vi "VNA and Keithlay 2400.vi"() -> ()   [LabVIEW 2022 SP3]
uses:
  <instrlib>/Keithley 24XX/Public/Data/Read (Single Point).vi
  <vilib>/Utility/file.llb/Write Delimited Spreadsheet (DBL).vi
  <instrlib>/Keithley 24XX/Keithley 24XX.lvlib
  Agilent ENA Series/Agilent ENA Series.lvlib
panel:
  out "Numeric 3":dbl
  in  "Numeric 2":dbl
  in  "Numeric":i32
  out "Status":sgl
  out "Current":sgl
  out "XY Graph":cluster{dbl[], "Primary / Real":dbl[]}(graph)
  out "Step V":dbl
  in  "Points (>1) V":u32=66
  in  "End V":dbl
  in  "Start V":dbl=-3.0
  in  "VNA VISA resource name":refnum<visa-resource-name>="E5061A"
  in  "Port ( 1)":i32=1
  in  "Measurement Parameters":u16(ring)=1 items=["S11", "S21", "S31", "S41", "S12", "S22", "S32", "S42", "S13", "S23", "S33", "S43", "S14", "S24", "S34", "S44", "A", "B", "C", "D", "R1", "R2", "R3", "R4"]
  in  "Power Level (dBm)":dbl=-5.0 format="%^.2g"
  in  "VNA Points":i32=1000
  in  "Start (Mhz)":dbl=1.0 format="%^.2e"
  in  "Stop (MHz)":dbl=10.0 format="%^.2e"
  in  "Trigger Source":u16(ring) items=["Internal", "External", "Manual", "BUS"]
  in  "Point Trigger (F: Disable)":bool
  in  "Continuous Sweep (T: Enable)":bool=TRUE
  in  "Averaging State (F: Off)":bool
  in  "Average Factor (16)":i32=16
  in  "IF Bandwidth (100000.0)":dbl=1000.0 format="%^.1e"
  in  "Smoothing State (F: Off)":bool
  in  "Wait time (ms)":dbl=4000.0
  in  "file path (dialog if empty)":path=path "C:/Users/B1172_SHG/Documents/NOEMS/test.txt"
  in  "Output Type  (0: Immediate)":u16(ring) items=["Immediate", "Triggered"]
  in  "Source Mode  (0: Voltage)":u16(ring) items=["Voltage", "Current"]
  out "Current Voltage":dbl
  in  "Compliance  Level (0.1)":dbl=0.1
  in  "Keithley VISA resource name":refnum<visa-resource-name>
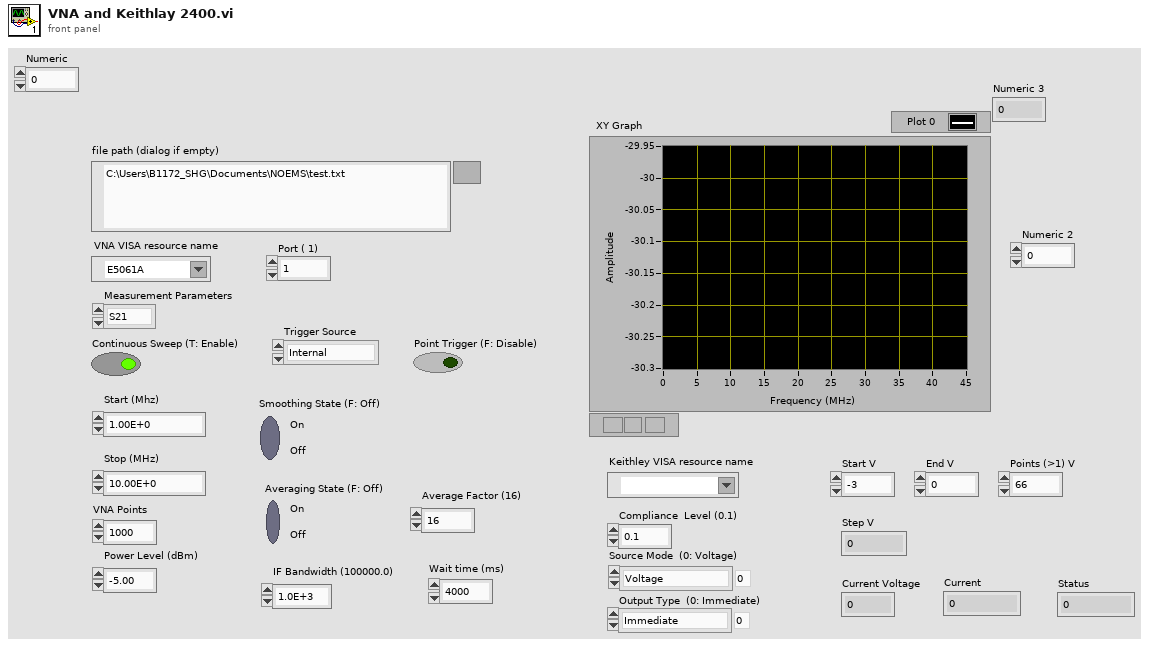
[diagram p1: front panel]
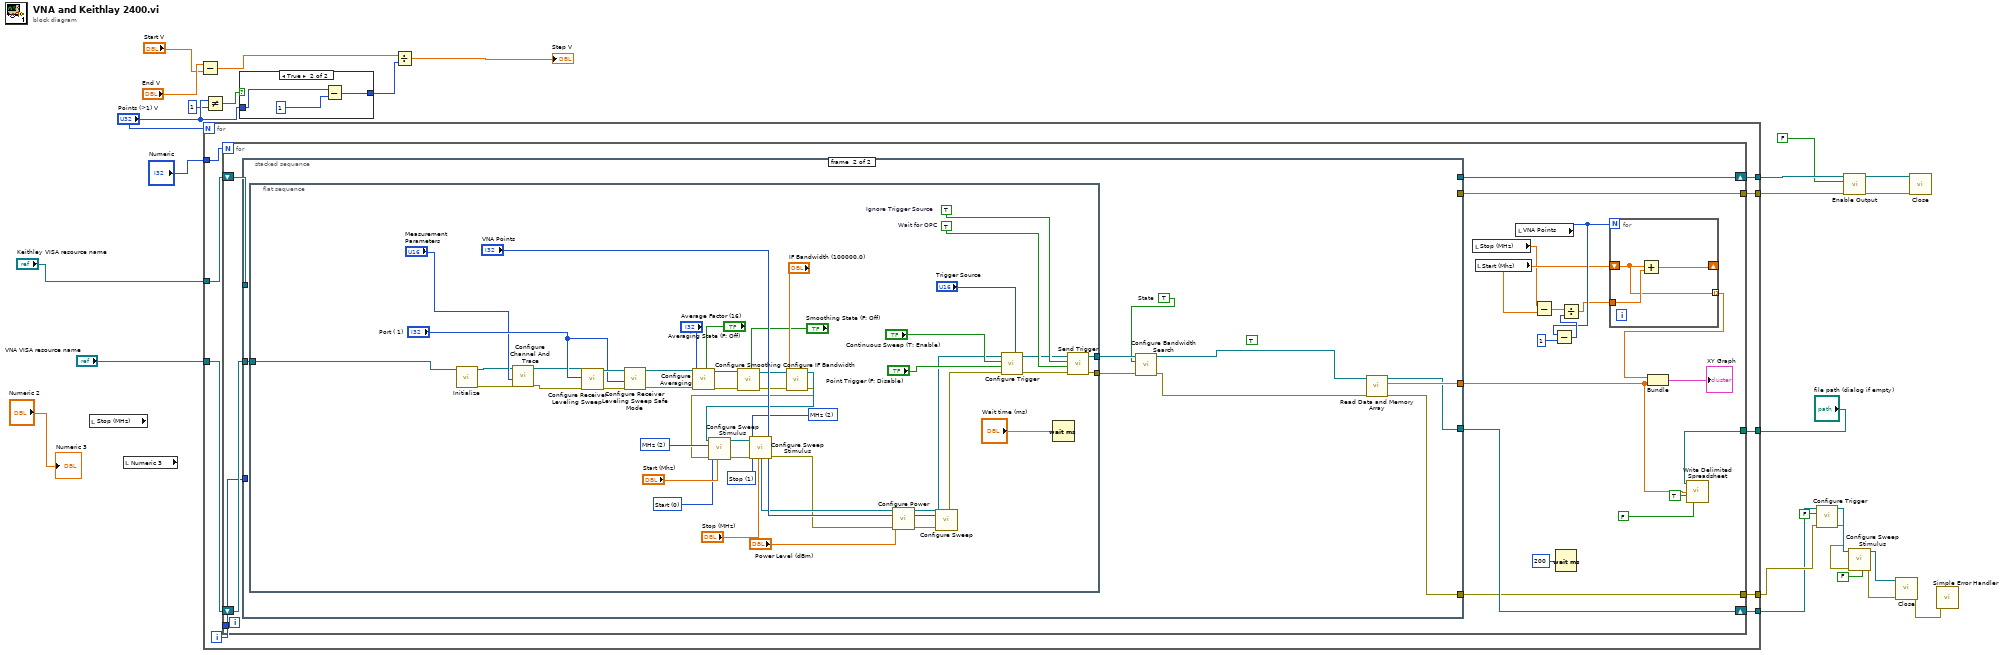
[diagram p0: block diagram]
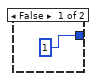
[diagram p2: hidden frame]
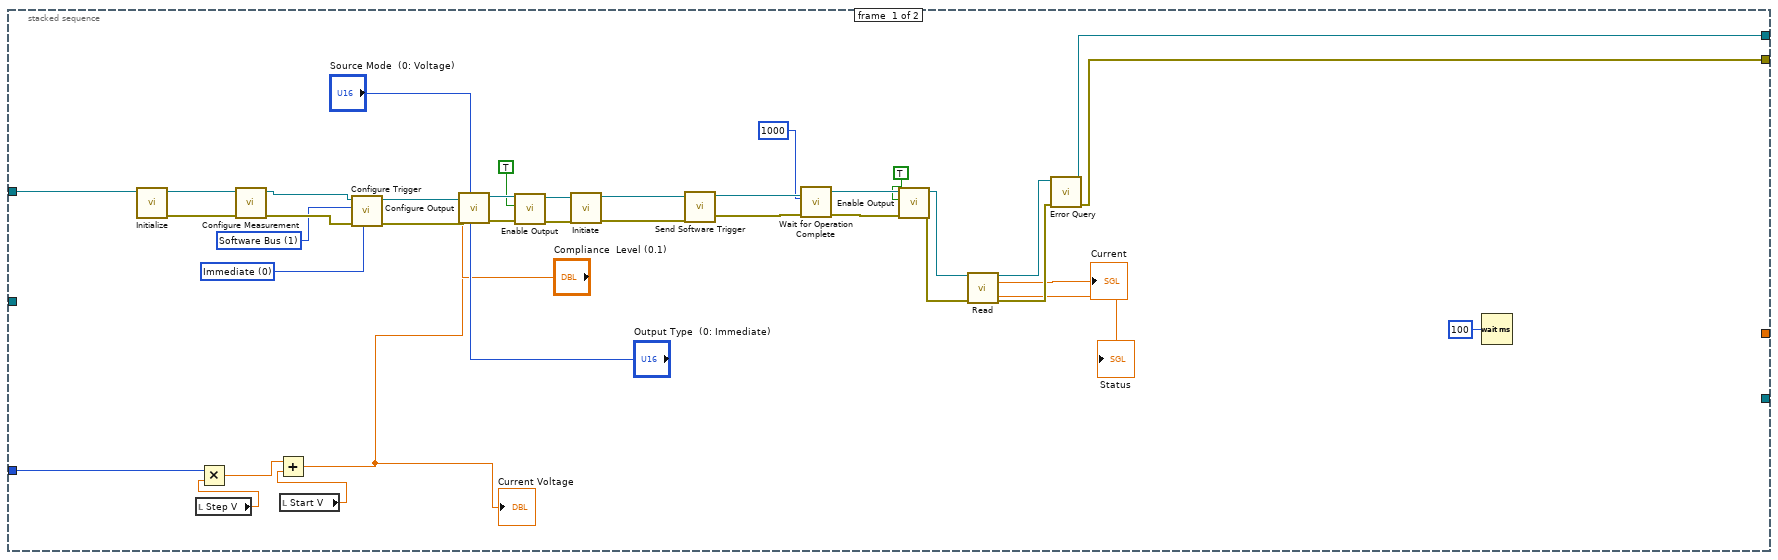
[diagram p3: hidden frame]
diagram:
  n1 = local read "Stop (MHz)"() -> ()  [unwired: 1 out]
  n2 = local read "Numeric 3"() -> ()  [unwired: 1 out]
  n3 = Subtract(x="End V", y="Start V") -> (x-y=w22:dbl)
  n4 = for {
    N: "Points (>1) V" -> [_]
    tunnel: "Keithley VISA resource name" -> [w36]
    tunnel: "VNA VISA resource name" -> [w35]
    tunnel: "file path (dialog if empty)" -> [w34]
    tunnel: [w32] -> w13
    tunnel: [w31] -> w15
    tunnel: [w30] -> w6
    tunnel: [w29] -> w7
    tunnel: "Numeric" -> [w28]
    i -> [w33]
    n5 = for {
      N: w28 -> [_]
      tunnel: w34 -> [w55]
      tunnel: w33 -> [w43]
      tunnel: [w42] -> w32
      tunnel: [w39] -> w29
      shift-right: [w41] -> w31
      shift-left: w36 -> [w57]
      shift-right: [w40] -> w30
      shift-left: w35 -> [w56]
      n6 = stacked-sequence {
        tunnel: w57 -> [w75 _]
        tunnel: w56 -> [_ w105]
        tunnel: w43 -> [w74 _]
        tunnel: [w69 _] -> w42
        tunnel: [w68 _] -> w41
        tunnel: [_ w100] -> w40
        tunnel: [_ w101] -> w39
        tunnel: [_ w103] -> w37
        frame #0 {
          w79 = u16 1 items=["Immediate", "Software Bus", "Timer", "Manual", "Trigger Link", "Rising SOT Pulse", "Falling SOT Pulse", "Rising or Falling SOT Pulse"] ("Arming Source  (0: Immediate)")
          w80 = u16 0 items=["Immediate", "Trigger Link"] ("Trigger Source (0: Immediate)")
          n7 = call <instrlib>:"Initialize.vi"("VISA resource name"=w75) -> ("error out"=w82:errorcluster, "VISA resource name out"=w81:refnum<visa-resource-name>)  [unwired: 9 in]
          n8 = local read "Step V"() -> (w73:dbl)
          n9 = Multiply(x=w74, y=w73) -> (x*y=w72:dbl)
          n10 = call <instrlib>:"Configure Measurement.vi"("error in (no error)"=w82, "VISA resource name"=w81) -> ("error out"=w99:errorcluster, "VISA resource name out"=w98:refnum<visa-resource-name>)  [unwired: 8 in]
          n11 = local read "Start V"() -> (w71:dbl)
          n12 = Add(x=w72, y=w71) -> (x+y=w70:dbl)
          "Current Voltage" <- w70
          n13 = call <instrlib>:"Configure Trigger.vi"("Trigger Source (0: Immediate)"=w80, "error in (no error)"=w99, "Arming Source  (0: Immediate)"=w79, "VISA resource name"=w98) -> ("error out"=w97:errorcluster, "VISA resource name out"=w96:refnum<visa-resource-name>)  [unwired: 6 in]
          n14 = call <instrlib>:"Configure Output.vi"("Output Type  (0: Immediate)"="Output Type  (0: Immediate)", "Source Mode  (0: Voltage)"="Source Mode  (0: Voltage)", "error in (no error)"=w97, "Compliance  Level (0.1)"="Compliance  Level (0.1)", "Output Level (0)"=w70, "VISA resource name"=w96) -> ("error out"=w84:errorcluster, "VISA resource name out"=w83:refnum<visa-resource-name>)  [unwired: 4 in]
          n15 = call <instrlib>:"Enable Output.vi"("error in (no error)"=w84, "Enable Output (T: Enable)"=TRUE, "VISA resource name"=w83) -> ("error out"=w86:errorcluster, "VISA resource name out"=w85:refnum<visa-resource-name>)  [unwired: 7 in]
          n16 = call <instrlib>:"Initiate.vi"("error in (no error)"=w86, "VISA resource name"=w85) -> ("error out"=w88:errorcluster, "VISA resource name out"=w87:refnum<visa-resource-name>)  [unwired: 8 in]
          n17 = call <instrlib>:"Send Software Trigger.vi"("error in (no error)"=w88, "VISA resource name"=w87) -> ("error out"=w93:errorcluster, "VISA resource name out"=w92:refnum<visa-resource-name>)  [unwired: 8 in]
          n18 = call <instrlib>:"Wait for Operation Complete.vi"("error in (no error)"=w93, "Timeout (10000 ms)"=u32 1000, "VISA resource name"=w92) -> ("error out"=w95:errorcluster, "VISA resource name out"=w94:refnum<visa-resource-name>)  [unwired: 7 in]
          n19 = call <instrlib>:"Enable Output.vi"("error in (no error)"=w95, "Enable Output (T: Enable)"=TRUE, "VISA resource name"=w94) -> ("error out"=w64:errorcluster, "VISA resource name out"=w66:refnum<visa-resource-name>)  [unwired: 7 in]
          n20 = call-poly <instrlib>:"Read.vi"("VISA resource name"=w66, "error in (no error)"=w64) -> ("VISA resource name out"=w65:refnum<visa-resource-name>, "Current"=→"Current":sgl, "Status"=→"Status":sgl, "error out"=w63:errorcluster)  [unwired: 7 in, 3 out]
          n21 = call <instrlib>:"Error Query.vi"("error in (no error)"=w63, "VISA resource name"=w65) -> ("error out"=w69:errorcluster, "VISA resource name out"=w68:refnum<visa-resource-name>)  [unwired: 6 in, 2 out]
          n22 = Wait (ms)(milliseconds to wait=u32 100) -> ()  [unwired: 1 out]
        }
        frame #1 {
          w107 = TRUE  # State
          (unwired) TRUE ("Continuous Sweep (T: Enable)")
          n23 = flat-sequence {
            tunnel: [w153] -> w108
            tunnel: [w111] -> w106
            tunnel: w105 -> [w109]
            frame #0 {
              w138 = u16 2 items=["Hz", "kHz", "MHz", "GHz", "dBm", "s", "V"] ("Unit (0: Hz)")
              w139 = u16 2 items=["Hz", "kHz", "MHz", "GHz", "dBm", "s", "V"] ("Unit (0: Hz)")
              w140 = u16 1 items=["Start", "Stop", "Center", "Span"] ("Stimulus (0: Start)")
              w141 = u16 0 items=["Start", "Stop", "Center", "Span"] ("Stimulus (0: Start)")
              w154 = TRUE  # Wait for OPC
              w155 = TRUE  # Ignore Trigger Source
              n24 = call <instrlib>:"Initialize.vi"("VISA resource name"=w109) -> ("error out"=w123:errorcluster, "VISA resource name out"=w127:refnum<visa-resource-name>)  [unwired: 9 in]
              n25 = call "Configure Channel And Trace.vi"("error in (no error)"=w123, "Measurement Parameters (0: S11)"="Measurement Parameters", "VISA resource name"=w127) -> ("error out"=w122:errorcluster, "VISA resource name out"=w126:refnum<visa-resource-name>)  [unwired: 7 in]
              n26 = call "Configure Receiver Leveling Sweep.vi"("VISA resource name"=w126, "Port ( 1)"="Port ( 1)", "error in (no error)"=w122) -> ("VISA resource name out"=w151:refnum<visa-resource-name>, "error out"=w121:errorcluster)  [unwired: 15 in]
              n27 = call "Configure Receiver Leveling Sweep Safe Mode.vi"("error in (no error)"=w121, "Port ( 1)"="Port ( 1)", "VISA resource name"=w151) -> ("error out"=w120:errorcluster, "VISA resource name out"=w125:refnum<visa-resource-name>)  [unwired: 7 in]
              n28 = call <instrlib>:"Configure Averaging.vi"("Averaging State (F: Off)"="Averaging State (F: Off)", "error in (no error)"=w120, "Factor (16)"="Average Factor (16)", "VISA resource name"=w125) -> ("error out"=w119:errorcluster, "VISA resource name out"=w134:refnum<visa-resource-name>)  [unwired: 6 in]
              n29 = call <instrlib>:"Configure Smoothing.vi"("Smoothing State (F: Off)"="Smoothing State (F: Off)", "error in (no error)"=w119, "VISA resource name"=w134) -> ("error out"=w118:errorcluster, "VISA resource name out"=w133:refnum<visa-resource-name>)  [unwired: 7 in]
              n30 = call <instrlib>:"Configure IF Bandwidth.vi"("error in (no error)"=w118, "IF Bandwidth (100000.0)"="IF Bandwidth (100000.0)", "VISA resource name"=w133) -> ("error out"=w117:errorcluster, "VISA resource name out"=w132:refnum<visa-resource-name>)  [unwired: 7 in]
              n31 = call "Configure Sweep Stimulus.vi"("Parameter (0.0)"="Start (Mhz)", "error in (no error)"=w117, "Stimulus (0: Start)"=w141, "Unit (0: Hz)"=w139, "VISA resource name"=w132) -> ("error out"=w116:errorcluster, "VISA resource name out"=w145:refnum<visa-resource-name>)  [unwired: 5 in]
              n32 = call "Configure Sweep Stimulus.vi"("Parameter (0.0)"="Stop (MHz)", "error in (no error)"=w116, "Stimulus (0: Start)"=w140, "Unit (0: Hz)"=w138, "VISA resource name"=w145) -> ("error out"=w115:errorcluster, "VISA resource name out"=w144:refnum<visa-resource-name>)  [unwired: 5 in]
              n33 = call "Configure Power.vi"("VISA resource name"=w144, "Power Level (0.0)"="Power Level (dBm)", "error in (no error)"=w115) -> ("VISA resource name out"=w147:refnum<visa-resource-name>, "error out"=w114:errorcluster)  [unwired: 11 in]
              n34 = call "Configure Sweep.vi"("VISA resource name"=w147, "Number of Measurement Points (201)"="VNA Points", "error in (no error)"=w114) -> ("VISA resource name out"=w124:refnum<visa-resource-name>, "error out"=w113:errorcluster)  [unwired: 11 in]
              n35 = call <instrlib>:"Configure Trigger.vi"("Trigger Source (0: Internal)"="Trigger Source", "error in (no error)"=w113, "Point Trigger (F: Disable)"="Point Trigger (F: Disable)", "Continuous Sweep (T: Enable)"="Continuous Sweep (T: Enable)", "VISA resource name"=w124) -> ("error out"=w112:errorcluster, "VISA resource name out"=w152:refnum<visa-resource-name>)  [unwired: 5 in]
              n36 = Wait (ms)(milliseconds to wait="Wait time (ms)") -> ()  [unwired: 1 out]
              n37 = call "Send Trigger.vi"("error in (no error)"=w112, "Wait for OPC (F: Do not Wait)"=w154, "Ignore Trigger Source (F: Do not Ignore)"=w155, "VISA resource name"=w152) -> ("error out"=w111:errorcluster, "VISA resource name out"=w153:refnum<visa-resource-name>)  [unwired: 6 in]
            }
          }
          n38 = call "Configure Bandwidth Search.vi"("error in (no error)"=w106, "Result Display State (F: Disable)"=w107, "VISA resource name"=w108) -> ("error out"=w102:errorcluster, "VISA resource name out"=w104:refnum<visa-resource-name>)  [unwired: 7 in]
          n39 = call "Read Data and Memory Array.vi"("error in (no error)"=w102, "VISA resource name"=w104) -> ("error out"=w101:errorcluster, "Primary / Real"=w103:dbl[], "VISA resource name out"=w100:refnum<visa-resource-name>)  [unwired: 6 in, 1 out]
        }
      }
      n40 = local read "Stop (MHz)"() -> (w47:dbl)
      n41 = local read "Start (Mhz)"() -> (w48:dbl)
      n42 = local read "VNA Points"() -> (w51:i32)
      n43 = Subtract(x=w47, y=w48) -> (x-y=w49:dbl)
      n44 = Subtract(x=w51, y=1) -> (x-y=w52:i32)
      n45 = Wait (ms)(milliseconds to wait=u32 200) -> ()  [unwired: 1 out]
      n46 = Divide(x=w49, y=w52) -> (x/y=w50:dbl)
      n47 = for {
        N: w51 -> [_]
        shift-right: [w60] -> _
        shift-left: w48 -> [w58]
        tunnel: w50 -> [w59]
        tunnel: [w58] -> w45 mode=indexing
        n48 = Add(x=w58, y=w59) -> (x+y=w60:dbl)
      }
      n49 = Bundle(w45, "Primary / Real"=w37) -> (→"XY Graph":cluster{dbl[], "Primary / Real":dbl[]})  [unwired: 1 in]
      n50 = call-poly <vilib>:"Write Delimited Spreadsheet.vi"("file path (dialog if empty)"=w55, "1D data"=w37, "append to file? (new file:F)"=TRUE, "transpose? (no:F)"=FALSE) -> ()  [unwired: 10 in, 2 out]
    }
  }
  n51 = Not Equal?(x="Points (>1) V", y=u32 1) -> (x != y?=w18:bool)
  n52 = case shown="True" w18 {
    tunnel: [1 w158] -> w20
    tunnel: "Points (>1) V" -> [_ w157]
    frame False {
    }
    frame True {
      n53 = Subtract(x=w157, y=u32 1) -> (x-y=w158:u32)
    }
  }
  n54 = Divide(x=w22, y=w20) -> (x/y=→"Step V":dbl)
  n55 = call <instrlib>:"Configure Trigger.vi"("error in (no error)"=w7, "Continuous Sweep (T: Enable)"=FALSE, "VISA resource name"=w6) -> ("error out"=w4:errorcluster, "VISA resource name out"=w5:refnum<visa-resource-name>)  [unwired: 7 in]
  n56 = call <instrlib>:"Enable Output.vi"("error in (no error)"=w13, "Enable Output (T: Enable)"=FALSE, "VISA resource name"=w15) -> ("error out"=w12:errorcluster, "VISA resource name out"=w14:refnum<visa-resource-name>)  [unwired: 7 in]
  n57 = call "Configure Sweep Stimulus.vi"("Signal Output (T: On)"=FALSE, "error in (no error)"=w4, "VISA resource name"=w5) -> ("error out"=w9:errorcluster, "VISA resource name out"=w10:refnum<visa-resource-name>)  [unwired: 7 in]
  n58 = call "Close.vi"("error in (no error)"=w9, "VISA resource name"=w10) -> ("error out"=w16:errorcluster)  [unwired: 9 in]
  n59 = call "Close.vi"("error in (no error)"=w12, "VISA resource name"=w14) -> ()  [unwired: 9 in, 1 out]
  n60 = call <vilib>:"Simple Error Handler.vi"("error in (no error)"=w16) -> ()  [unwired: 4 in, 5 out]
  "Numeric 3" <- "Numeric 2"
